vi "Parameters_Get_Mode.vi"(8 "error in (no error)":errorcluster, 10 "Parameters":dbl[](array[numeric])) -> (0 "error out":errorcluster, 2 "Parameters Out":dbl[](array[numeric]), 3 "Move Mode":T1=enum."Skip")   [LabVIEW 2017, in "WordManipulationLibrary.lvlib"]
uses:
  WordManipulationLibrary.lvlib
  MoveMode.ctl
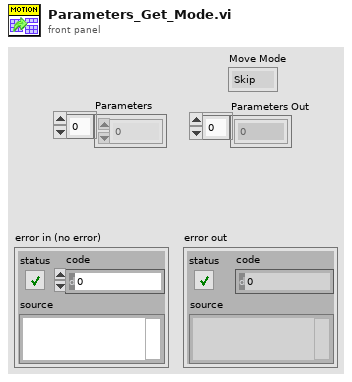
[diagram p1: front panel]
types:
  T1 = typedef "WordManipulationLibrary.lvlib/MoveMode.ctl" = enum16{"Reserved", "Profile Position Mode", "Velocity Mode", "Profile Velocity Mode", "Profile Torque Mode", "Reserved 2", "Reference Mode", "Interpolated Position Mode", "Skip"}
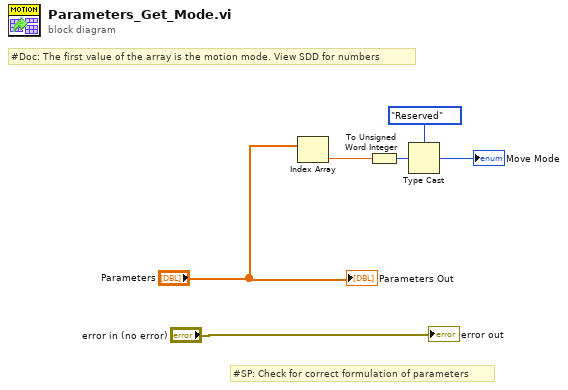
[diagram p0: block diagram]
diagram:
  # "#Doc: The first value of the array is the motion mode. View SDD for numbers"
  # "#SP: Check for correct formulation of parameters"
  n1 = Index Array(array="Parameters") -> (element=w5:dbl)  [unwired: 1 in]
  n2 = To Unsigned Word Integer(number=w5) -> (unsigned 16bit integer=w6:u16)
  n3 = Type Cast(type=MoveMode."Reserved" ("f"), x=w6) -> (*(type *) &x=→"Move Mode":T1)
  "Parameters Out" <- "Parameters"
  "error out" <- "error in (no error)"
